vi "CompareChkTime.vi"(9 "ChkUpdateCnt":refnum<vi>, 10 "LastTimChkUpdate":dbl, 11 "ChkUpdatePeriod":u32) -> (3 "OK2Chk":bool)   [LabVIEW 2015]
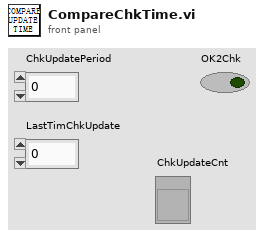
[diagram p1: front panel]
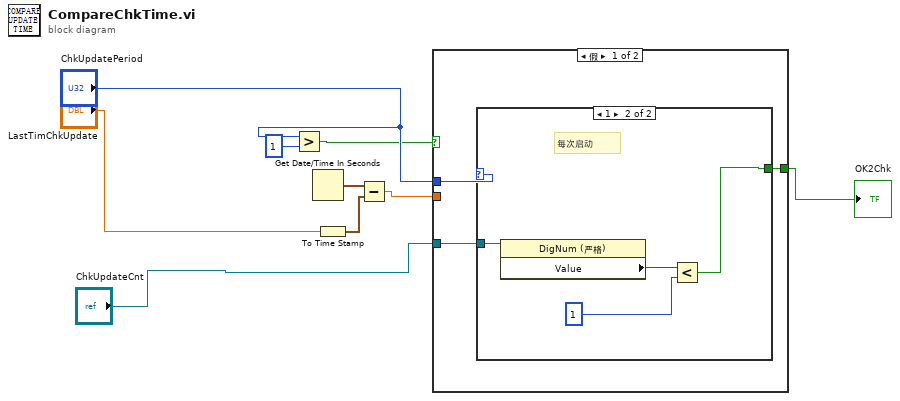
[diagram p0: block diagram]
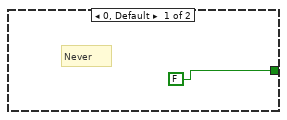
[diagram p2: hidden frame]
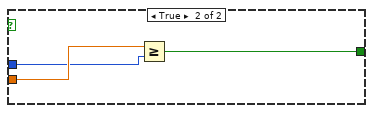
[diagram p3: hidden frame]
diagram:
  n1 = Greater?(x="ChkUpdatePeriod", y=u32 1) -> (0:w4:bool)
  n2 = Get Date/Time In Seconds() -> (seconds since 1Jan1904=w8:timestamp)
  n3 = To Time Stamp(1:"LastTimChkUpdate") -> (0:w9:timestamp)
  n4 = Subtract(x=w8, y=w9) -> (x-y=w2:dbl)
  n5 = case shown="假" w4 {
    tunnel: "ChkUpdatePeriod" -> [w12 w19]
    tunnel: w2 -> [_ w20]
    tunnel: [w11 w18] -> w3
    tunnel: "ChkUpdateCnt" -> [w10 _]
    frame False {
      n6 = case shown="1" w12 {
        tunnel: [FALSE w14] -> w11
        tunnel: w10 -> [_ w15]
        frame 0, Default {
          # "Never"
        }
        frame 1 {
          # "每次启动"
          n7 = property class="DigNum (严格)"(reference=w15) -> ("Value"=w16:i32)  [unwired: 1 in, 2 out]
          n8 = Less?(x=w16, y=1) -> (x < y?=w14:bool)
        }
      }
    }
    frame True {
      n9 = Greater Or Equal?(x=w20, y=w19) -> (x >= y?=w18:bool)
    }
  }
  "OK2Chk" <- w3
